vi "FM_RecieverLogic.vi"(8 "SampleFrequencyHz":dbl=2.5, 9 "Tuner in":dbl=102.367, 10 "CarrierFrequencyHz":dbl=102.1, 11 "Data in":cdb[](array[numeric])=array[125000 elements]) -> (1 "FFT":cluster{"f0":dbl, "df":dbl, "magnitude":dbl[]}, 3 "Audio":dbl[](array[numeric]))   [LabVIEW 2020]
uses:
  <vilib>/Analysis/3filter.llb/Filter Passband Type.ctl
  <vilib>/Analysis/3filter.llb/Elliptic Filter (DBL).vi
  <vilib>/Analysis/NI_AALPro.lvlib
  <vilib>/Analysis/NI_AALBase.lvlib
  <vilib>/Analysis/2dsp.llb/Complex FFT.vi
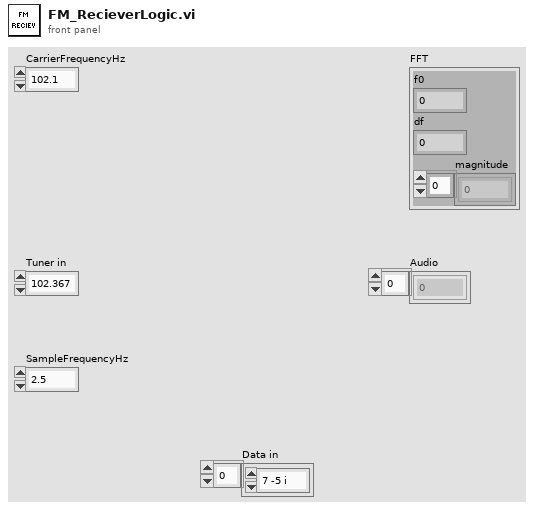
[diagram p1: front panel]
types:
  T1 = typedef "NI_AALBase.lvlib/Filter Passband Type.ctl" = enum32{"Lowpass", "Highpass", "Bandpass", "Bandstop"}
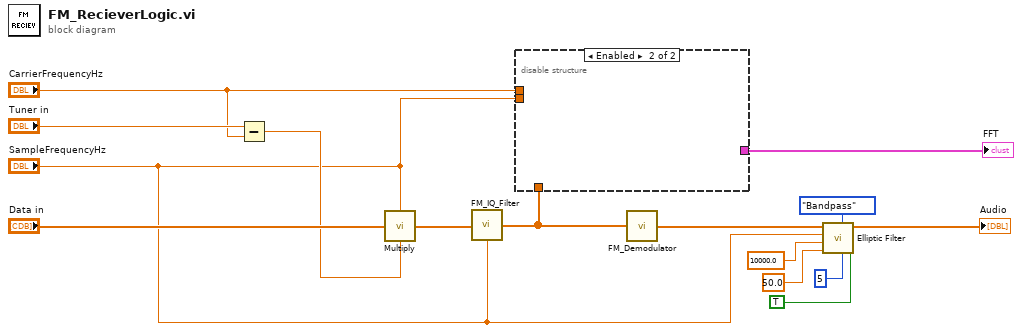
[diagram p0: block diagram]
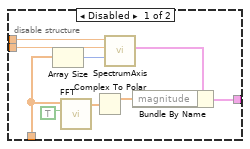
[diagram p2: hidden frame]
diagram:
  n1 = Subtract(x="Tuner in", y="CarrierFrequencyHz") -> (x-y=w5:dbl)
  n2 = call "Multiply.vi"("SampleFreq"="SampleFrequencyHz", "Array in"="Data in", "MultiplyFreq"=w5) -> ("Array out"=w4:cdb[])  [unwired: 12 in]
  n3 = call "FM_IQ_Filter.vi"("Sample freq"="SampleFrequencyHz", "Array in"=w4) -> ("Array"=w3:cdb[])  [unwired: 13 in]
  n4 = disable-structure shown="Enabled" {
    disable-tunnel: [w24 _] -> w15
    disable-tunnel: "CarrierFrequencyHz" -> [w23 _]
    disable-tunnel: w3 -> [w17 _]
    disable-tunnel: "SampleFrequencyHz" -> [w16 _]
    frame Disabled {
      n5 = Array Size(array=w17) -> (size(s)=w22:i32)
      n6 = call-poly <vilib>:"FFT.vi"("shift?"=TRUE, "X"=w17) -> ("FFT {X}"=w18:cdb[])  [unwired: 8 in, 1 out]
      n7 = Complex To Polar(r * e^(i*theta)=w18) -> (r=w20:dbl[])  [unwired: 1 out]
      n8 = call "SpectrumAxis.vi"("FFT Size"=w22, "SampleFreq"=w16, "CarrierFreqz)"=w23) -> ("SpectrumConstant"=w21:cluster{"f0":dbl, "df":dbl, "magnitude":dbl[]})  [unwired: 8 in]
      n9 = Bundle By Name(cluster=w21, "magnitude"=w20) -> (w24:cluster{"f0":dbl, "df":dbl, "magnitude":dbl[]})
    }
    frame Enabled {
    }
  }
  "FFT" <- w15
  n10 = call "FM_Demodulator.vi"("Array in"=w3) -> ("Array out"=w2:dbl[])
  n11 = call-poly <vilib>:"Elliptic Filter.vi"("init/cont (init:F)"=TRUE, "order"=5, "filter type"=Filter_Passband_Type."Bandpass", "low cutoff freq: fl"=50.0, "high cutoff freq: fh"=10000.0, "sampling freq: fs"="SampleFrequencyHz", "X"=w2) -> ("Filtered X"=→"Audio":dbl[])  [unwired: 3 in, 1 out]
